vi "Parse Object.vi"(8 "error in (no error)":errorcluster, 10 "Index In":i32, 11 "JSON String":string) -> (0 "error out":errorcluster, 2 "Index Out":i32, 3 "JSON Value out":variant)   [LabVIEW 2017, in "Advanced Variant Tools.lvlib" / "JSON.lvlib"]
uses:
  JSON/JSON.lvlib
  Errors.ctl
  Token Type.ctl
  Cluster Manipulation/Data Manipulation.lvlib
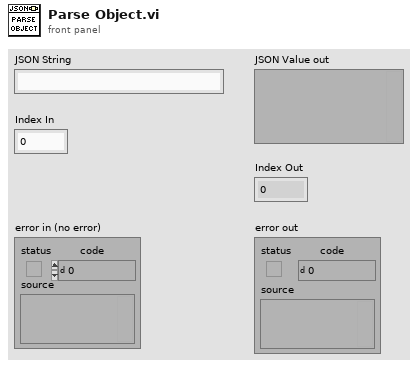
[diagram p1: front panel]
types:
  T1 = typedef "Advanced Variant Tools.lvlib/JSON.lvlib/Errors.ctl" = enum16{"No key", "Key path type", "Array OOB", "Type Mismatch", "Invalid Token", "Invalid Value"}
  T2 = typedef "Advanced Variant Tools.lvlib/JSON.lvlib/Token Type.ctl" = enum16{"NONE", "CURLY_OPEN", "CURLY_CLOSE", "SQUARED_OPEN", "SQUARED_CLOSE", "COLON", "COMMA", "STRING", "NUMBER", "TRUE", "FALSE", "NULL"}
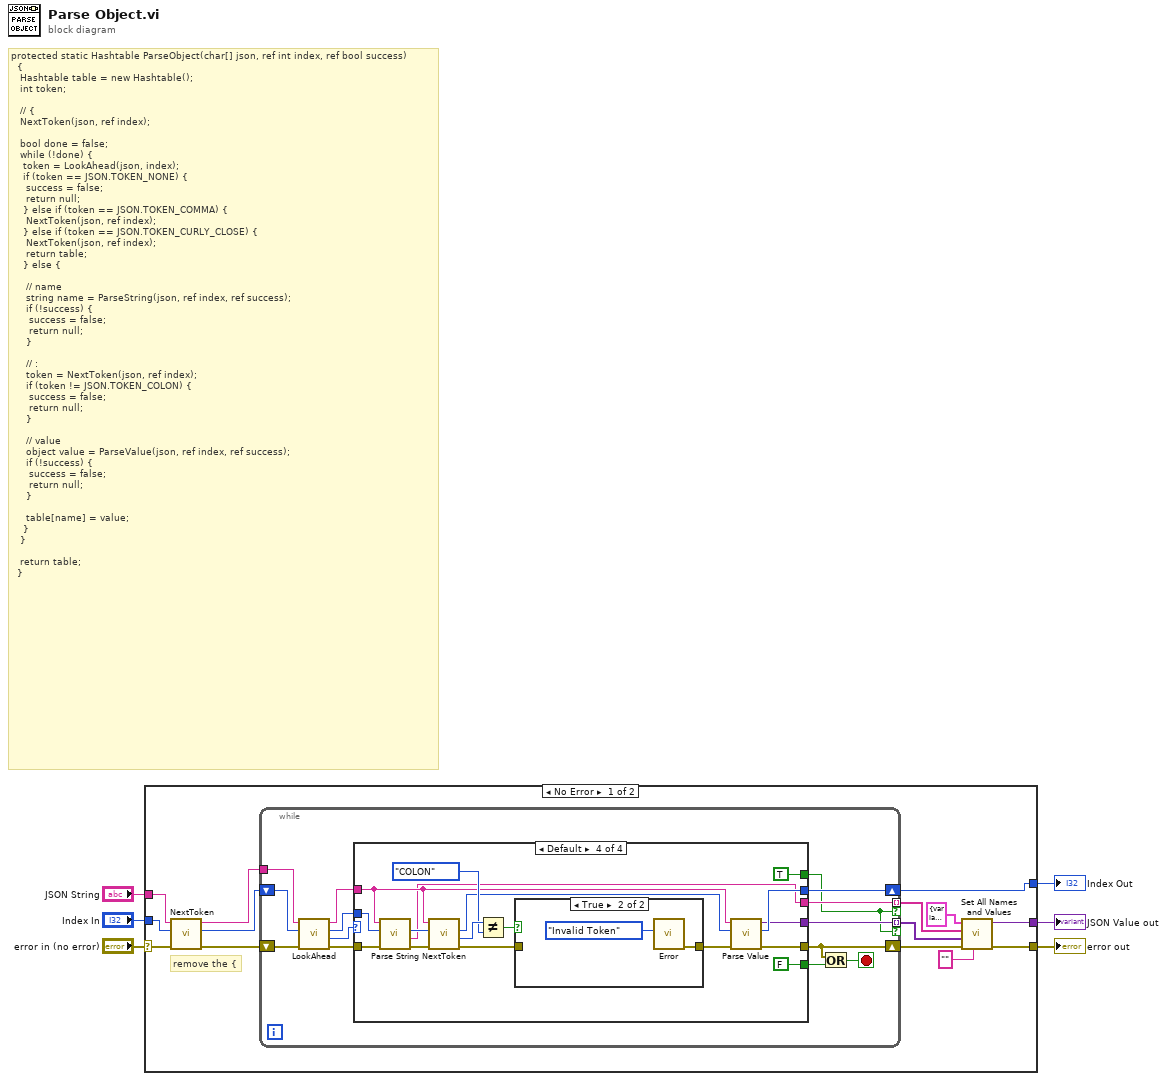
[diagram p0: block diagram]
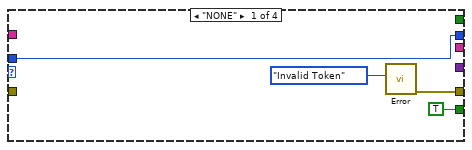
[diagram p2: hidden frame]
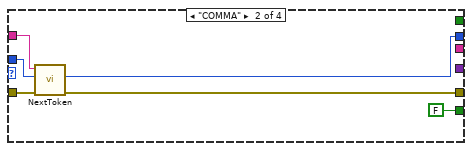
[diagram p3: hidden frame]
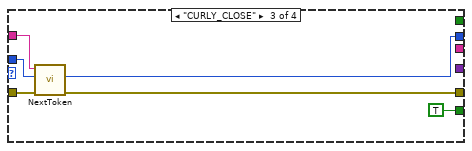
[diagram p4: hidden frame]
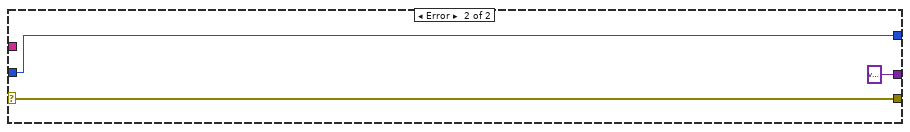
[diagram p6: hidden frame]
diagram:
  # "protected static Hashtable ParseObject(char[] json, ref int index, ref bool success)\n\t\t{\n\t\t\tHashtable table = new Hashtable();\n\t\t\tint token;\n\n\t\t\t// {\n\t\t\tNextToken(json, ref index);\n\n\t\t\tbool done = false;\n\t\t\twhile (!done) {\n\t\t\t\ttoken = LookAhead(json, index);\n\t\t\t\tif (token == JSON.TOKEN_NONE) {\n\t\t\t\t\tsuccess = false;\n\t\t\t\t\treturn null;\n\t\t\t\t} else if (token == JSON.TOKEN_COMMA) {\n\t\t\t\t\tNextToken(json, ref index);\n\t\t\t\t} else if (token == JSON.TOKEN_CURLY_CLOSE) {\n\t\t\t\t\tNextToken(json, ref index);\n\t\t\t\t\treturn table;\n\t\t\t\t} else {\n\n\t\t\t\t\t// name\n\t\t\t\t\tstring name = ParseString(json, ref index, ref success);\n\t\t\t\t\tif (!success) {\n\t\t\t\t\t\tsuccess = false;\n\t\t\t\t\t\treturn null;\n\t\t\t\t\t}\n\n\t\t\t\t\t// :\n\t\t\t\t\ttoken = NextToken(json, ref index);\n\t\t\t\t\tif (token != JSON.TOKEN_COLON) {\n\t\t\t\t\t\tsuccess = false;\n\t\t\t\t\t\treturn null;\n\t\t\t\t\t}\n\n\t\t\t\t\t// value\n\t\t\t\t\tobject value = ParseValue(json, ref index, ref success);\n\t\t\t\t\tif (!success) {\n\t\t\t\t\t\tsuccess = false;\n\t\t\t\t\t\treturn null;\n\t\t\t\t\t}\n\n\t\t\t\t\ttable[name] = value;\n\t\t\t\t}\n\t\t\t}\n\n\t\t\treturn table;\n\t\t}"
  n1 = case shown="No Error" "error in (no error)" {
    selector: "error in (no error)" -> [w16 w72]
    tunnel: [w10 w72] -> w5
    tunnel: "Index In" -> [w17 w73]
    tunnel: [w20 w73] -> w3
    tunnel: [w11 variant ("VCluster")] -> w1
    tunnel: "JSON String" -> [w14 _]
    frame No Error {
      # "remove the {"
      n2 = call "NextToken.vi"("error in (no error)"=w16, "Index In"=w17, "JSON String"=w14) -> ("error out"=w19:errorcluster, "Index Out"=w18:i32, "JSON String Passthrough"=w15:string)  [unwired: 5 in, 1 out]
      n3 = while {
        tunnel: w15 -> [w33]
        shift-right: [w28] -> w20
        shift-left: w18 -> [w32]
        shift-right: [w24] -> w9
        shift-left: w19 -> [w34]
        tunnel: [w23] -> w12 mode=indexing if=w21
        tunnel: [w22] -> w8 mode=indexing if=w21
        stop <- w25 stop-if-true
        n4 = call "LookAhead.vi"("error in (no error)"=w34, "Index"=w32, "JSON String"=w33) -> ("error out"=w30:errorcluster, "TOKEN"=w31:T2, "Index Passthrough"=w29:i32, "JSON String Passthrough"=w27:string)  [unwired: 5 in]
        n5 = case shown="Default" w31 {
          tunnel: [TRUE FALSE TRUE FALSE] -> w26
          tunnel: w30 -> [_ w44 w50 w67]
          tunnel: [w36 w41 w47 w58] -> w24
          tunnel: w29 -> [w37 w43 w49 w66]
          tunnel: [w37 w42 w48 w59] -> w28
          tunnel: w27 -> [_ w39 w45 w61]
          tunnel: [_ _ _ w53] -> w23
          tunnel: [_ _ _ w52] -> w22
          tunnel: [_ _ _ TRUE] -> w21
          frame "NONE" {
            n6 = call "Error.vi"(9:Errors."Invalid Token") -> ("error out"=w36:errorcluster)  [unwired: 9 in]
          }
          frame "COMMA" {
            n7 = call "NextToken.vi"("error in (no error)"=w44, "Index In"=w43, "JSON String"=w39) -> ("error out"=w41:errorcluster, "Index Out"=w42:i32)  [unwired: 5 in, 2 out]
          }
          frame "CURLY_CLOSE" {
            n8 = call "NextToken.vi"("error in (no error)"=w50, "Index In"=w49, "JSON String"=w45) -> ("error out"=w47:errorcluster, "Index Out"=w48:i32)  [unwired: 5 in, 2 out]
          }
          frame Default {
            n9 = call "Parse String.vi"("error in (no error)"=w67, "Index In"=w66, "JSON String"=w61) -> ("error out"=w65:errorcluster, "Parsed String"=w53:string, "Index Out"=w64:i32)  [unwired: 5 in, 1 out]
            n10 = call "NextToken.vi"("error in (no error)"=w65, "Index In"=w64, "JSON String"=w61) -> ("error out"=w54:errorcluster, "TOKEN"=w63:T2, "Index Out"=w60:i32)  [unwired: 5 in, 1 out]
            n11 = Not Equal?(x=w63, y=Token_Type."COLON") -> (x != y?=w56:bool)
            n12 = case shown="True" w56 {
              tunnel: [w68 w69] -> w55
              tunnel: w54 -> [w68 _]
              frame False {
              }
              frame True {
                n13 = call "Error.vi"(9:Errors."Invalid Token") -> ("error out"=w69:errorcluster)  [unwired: 9 in]
              }
            }
            n14 = call "Parse Value.vi"("error in (no error)"=w55, "Index In"=w60, "JSON String"=w61) -> ("error out"=w58:errorcluster, "Index Out"=w59:i32, "JSON Value out"=w52:variant)  [unwired: 6 in]
          }
        }
        n15 = Or(x=w24, y=w26) -> (x .or. y?=w25:bool)
      }
      n16 = call "Set All Names and Values.vi"("Name"="", "error in"=w9, "values"=w8, "Item Names"=w12, "Cluster In"=cluster{"Variant out":variant} {"Variant out"=variant}) -> ("error out"=w10:errorcluster, "Cluster Out"=w11:variant)  [unwired: 5 in]
    }
    frame Error {
    }
  }
  "error out" <- w5
  "Index Out" <- w3
  "JSON Value out" <- w1
